vi "Expand Key.vi"(1 "Mode (auto)":enum16{"128", "192", "256", "auto"}(ring)=enum."auto", 7 "Key":u32[](array[numeric])=[49, 0, 0, 0, 0, 0, 0, 0, 0, 0, 0, 0, 0, 0, 0, 0, 0, 0, 0, 0, 0, 0, 0, 0, 0, 0, 0, 0, 0, 0, 0, 0], 11 "error in":errorcluster) -> (8 "Expanded Key":u32[](array[numeric]), 15 "error out":errorcluster)   [LabVIEW 2020, in "Library Commun.lvlib" / "Advanced Encryption Standard (AES).lvlib"]
doc: "The function KeyExpansion() supplies a much expanded (and transformed) key for use by the AddRoundKey() function in the main AES algorithm. In the case of the AES, there are a number of rounds, each needing its own key, so the actual key is ''stretched out'' and transformed to give portions of key for each round. This is the key expansion.\n\n<inline>"
uses:
  Advanced Encryption Standard (AES).lvlib
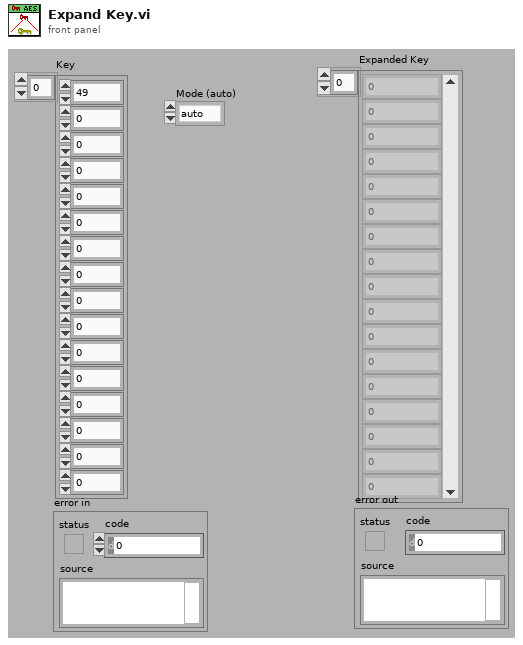
[diagram p1: front panel]
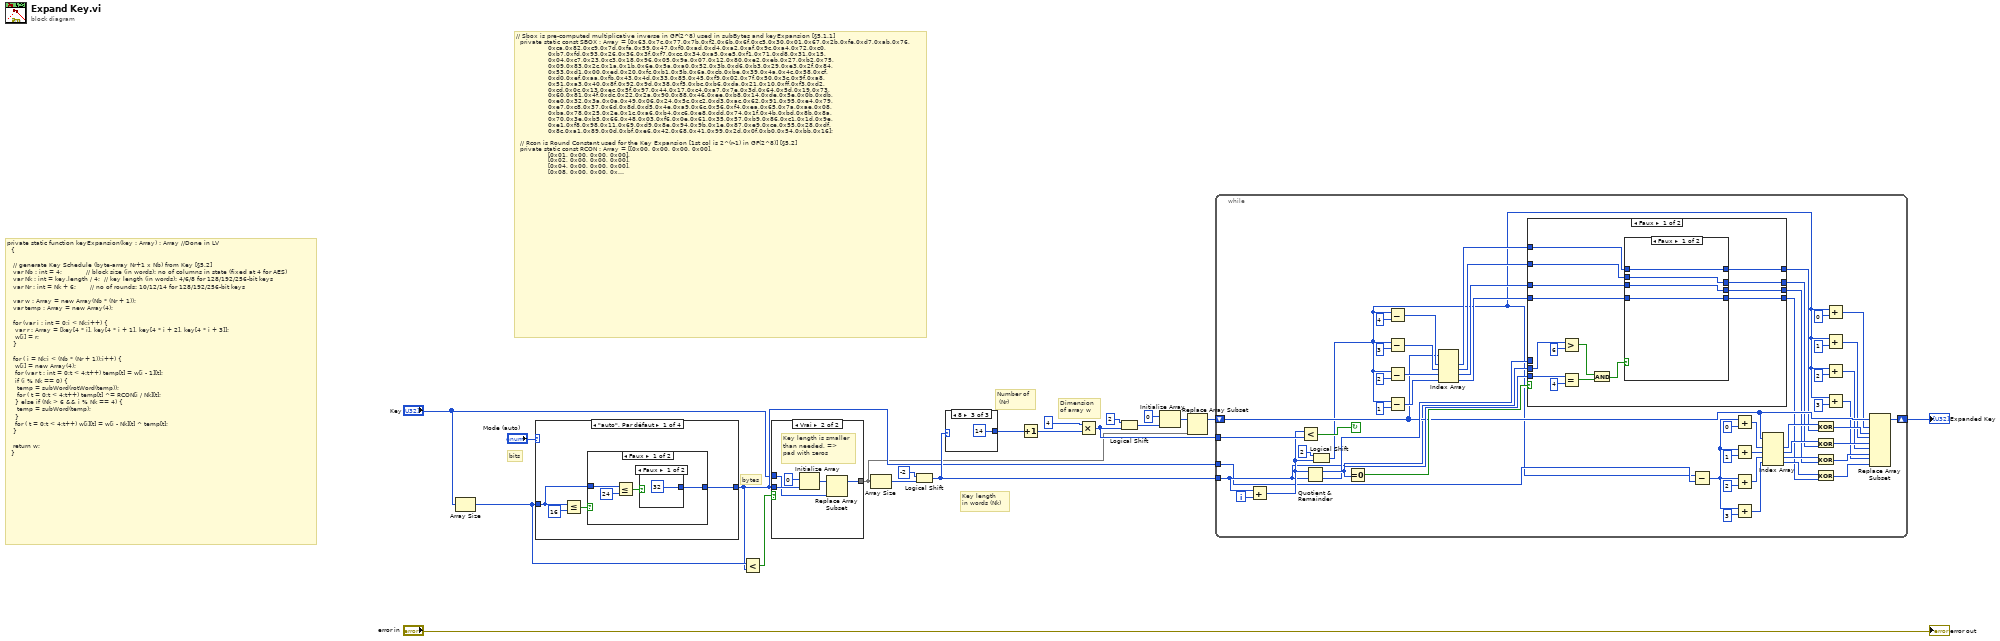
[diagram p0: block diagram]
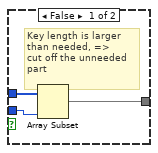
[diagram p2: hidden frame]
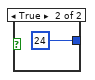
[diagram p3: hidden frame]
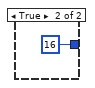
[diagram p4: hidden frame]
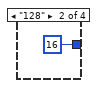
[diagram p5: hidden frame]
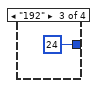
[diagram p6: hidden frame]
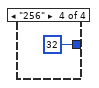
[diagram p7: hidden frame]
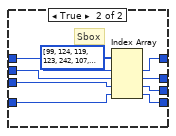
[diagram p8: hidden frame]
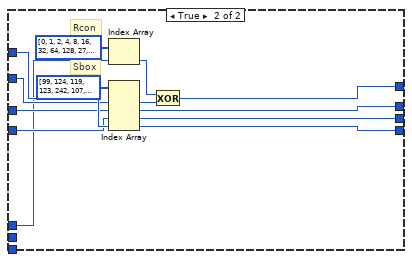
[diagram p9: hidden frame]
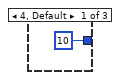
[diagram p10: hidden frame]
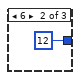
[diagram p11: hidden frame]
diagram:
  # "// Sbox is pre-computed multiplicative inverse in GF(2^8) used in subBytes and keyExpansion [§5.1.1]\n\t\tprivate static const SBOX : Array = [0x63,0x7c,0x77,0x7b,0xf2,0x6b,0x6f,0xc5,0x30,0x01,0x67,0x2b,0xfe,0xd7,0xab,0x76,\n\t\t\t             0xca,0x82,0xc9,0x7d,0xfa,0x59,0x47,0xf0,0xad,0xd4,0xa2,0xaf,0x9c,0xa4,0x72,0xc0,\n\t\t\t             0xb7,0xfd,0x93,0x26,0x36,0x3f,0xf7,0xcc,0x34,0xa5,0xe5,0xf1,0x71,0xd8,0x31,0x15,\n\t\t\t             0x04,0xc7,0x23,0xc3,0x18,0x96,0x05,0x9a,0x07,0x12,0x80,0xe2,0xeb,0x27,0xb2,0x75,\n\t\t\t             0x09,0x83,0x2c,0x1a,0x1b,0x6e,0x5a,0xa0,0x52,0x3b,0xd6,0xb3,0x29,0xe3,0x2f,0x84,\n\t\t\t             0x53,0xd1,0x00,0xed,0x20,0xfc,0xb1,0x5b,0x6a,0xcb,0xbe,0x39,0x4a,0x4c,0x58,0xcf,\n\t\t\t             0xd0,0xef,0xaa,0xfb,0x43,0x4d,0x33,0x85,0x45,0xf9,0x02,0x7f,0x50,0x3c,0x9f,0xa8,\n\t\t\t             0x51,0xa3,0x40,0x8f,0x92,0x9d,0x38,0xf5,0xbc,0xb6,0xda,0x21,0x10,0xff,0xf3,0xd2,\n\t\t\t             0xcd,0x0c,0x13,0xec,0x5f,0x97,0x44,0x17,0xc4,0xa7,0x7e,0x3d,0x64,0x5d,0x19,0x73,\n\t\t\t             0x60,0x81,0x4f,0xdc,0x22,0x2a,0x90,0x88,0x46,0xee,0xb8,0x14,0xde,0x5e,0x0b,0xdb,\n\t\t\t             0xe0,0x32,0x3a,0x0a,0x49,0x06,0x24,0x5c,0xc2,0xd3,0xac,0x62,0x91,0x95,0xe4,0x79,\n\t\t\t             0xe7,0xc8,0x37,0x6d,0x8d,0xd5,0x4e,0xa9,0x6c,0x56,0xf4,0xea,0x65,0x7a,0xae,0x08,\n\t\t\t             0xba,0x78,0x25,0x2e,0x1c,0xa6,0xb4,0xc6,0xe8,0xdd,0x74,0x1f,0x4b,0xbd,0x8b,0x8a,\n\t\t\t             0x70,0x3e,0xb5,0x66,0x48,0x03,0xf6,0x0e,0x61,0x35,0x57,0xb9,0x86,0xc1,0x1d,0x9e,\n\t\t\t             0xe1,0xf8,0x98,0x11,0x69,0xd9,0x8e,0x94,0x9b,0x1e,0x87,0xe9,0xce,0x55,0x28,0xdf,\n\t\t\t             0x8c,0xa1,0x89,0x0d,0xbf,0xe6,0x42,0x68,0x41,0x99,0x2d,0x0f,0xb0,0x54,0xbb,0x16];\n\n\t\t// Rcon is Round Constant used for the Key Expansion [1st col is 2^(r-1) in GF(2^8)] [§5.2]\n\t\tprivate static const RCON : Array = [[0x00, 0x00, 0x00, 0x00],\n\t\t\t             [0x01, 0x00, 0x00, 0x00],\n\t\t\t             [0x02, 0x00, 0x00, 0x00],\n\t\t\t             [0x04, 0x00, 0x00, 0x00],\n\t\t\t             [0x08, 0x00, 0x00, 0x00],\n\t\t\t             [0x10, 0x00, 0x00, 0x00],\n\t\t\t             [0x20, 0x00, 0x00, 0x00],\n\t\t\t             [0x40, 0x00, 0x00, 0x00],\n\t\t\t             [0x80, 0x00, 0x00, 0x00],\n\t\t\t             [0x1b, 0x00, 0x00, 0x00],\n\t\t\t             [0x36, 0x00, 0x00, 0x00]];"
  # "private static function keyExpansion(key : Array) : Array //Done in LV\n\t\t{  \n\t\t\t\n\t\t\t// generate Key Schedule (byte-array Nr+1 x Nb) from Key [§5.2]\n\t\t\tvar Nb : int = 4;            // block size (in words): no of columns in state (fixed at 4 for AES)\n\t\t\tvar Nk : int = key.length / 4;  // key length (in words): 4/6/8 for 128/192/256-bit keys\n\t\t\tvar Nr : int = Nk + 6;       // no of rounds: 10/12/14 for 128/192/256-bit keys\n\n\t\t\tvar w : Array = new Array(Nb * (Nr + 1));\n\t\t\tvar temp : Array = new Array(4);\n\t\t\t\n\t\t\tfor (var i : int = 0;i < Nk;i++) {\n\t\t\t\tvar r : Array = [key[4 * i], key[4 * i + 1], key[4 * i + 2], key[4 * i + 3]];\n\t\t\t\tw[i] = r;\n\t\t\t}\n\t\t\t\n\t\t\tfor ( i = Nk;i < (Nb * (Nr + 1));i++) {\n\t\t\t\tw[i] = new Array(4);\n\t\t\t\tfor (var t : int = 0;t < 4;t++) temp[t] = w[i - 1][t];\n\t\t\t\tif (i % Nk == 0) {\n\t\t\t\t\ttemp = subWord(rotWord(temp));\n\t\t\t\t\tfor ( t = 0;t < 4;t++) temp[t] ^= RCON[i / Nk][t];\n\t\t\t\t} else if (Nk > 6 && i % Nk == 4) {\n\t\t\t\t\ttemp = subWord(temp);\n\t\t\t\t}\n\t\t\t\tfor ( t = 0;t < 4;t++) w[i][t] = w[i - Nk][t] ^ temp[t];\n\t\t\t}\n\t\t\t\n\t\t\treturn w;\n\t\t}"
  # "Dimension \nof array w"
  # "Number of\n (Nr)"
  # "Key length \nin words (Nk)"
  # "bytes"
  # "bits"
  n1 = Array Size(array="Key") -> (size(s)=w7:i32)
  n2 = case shown="\"auto\", Par défaut" "Mode (auto)" {
    tunnel: w7 -> [w21 _ _ _]
    tunnel: [w22 16 24 32] -> w5
    frame "auto", Default {
      n3 = Less Or Equal?(x=w21, y=16) -> (x <= y?=w23:bool)
      n4 = case shown="Faux" w23 {
        tunnel: [w25 16] -> w22
        tunnel: w21 -> [w28 _]
        frame False {
          n5 = Less Or Equal?(x=w28, y=24) -> (x <= y?=w26:bool)
          n6 = case shown="Faux" w26 {
            tunnel: [32 ("y") 24 ("y")] -> w25
            frame False {
            }
            frame True {
            }
          }
        }
        frame True {
        }
      }
    }
    frame "128" {
    }
    frame "192" {
    }
    frame "256" {
    }
  }
  n7 = Less?(x=w7, y=w5) -> (x < y?=w6:bool)
  n8 = case shown="Vrai" w6 {
    tunnel: "Key" -> [w37 w38]
    tunnel: w5 -> [w36 w42]
    tunnel: [w35 w40] -> w4
    frame False {
      # "Key length is larger\nthan needed, =>\ncut off the unneeded\npart"
      n9 = Array Subset(array=w37, length=w36) -> (w35:u32[])  [unwired: 1 in]
    }
    frame True {
      # "Key length is smaller\nthan needed, =>\npad with zeros"
      n10 = Initialize Array(u32 0, w42) -> (w41:u32[])
      n11 = Replace Array Subset(array=w41, new element=w38) -> (w40:u32[])  [unwired: 1 in]
    }
  }
  n12 = Array Size(array=w4) -> (size(s)=w9:i32)
  n13 = Logical Shift(y=i8 -2, x=w9) -> (x << y=w16:i32)
  n14 = case shown="8" w16 {
    tunnel: [10 12 14] -> w19
    frame 4, Default {
    }
    frame 6 {
    }
    frame 8 {
    }
  }
  n15 = Increment(x=w19) -> (x+1=w18:i32)
  n16 = Multiply(x=4, y=w18) -> (x*y=w12:i32)
  n17 = Logical Shift(y=i8 2, x=w12) -> (x << y=w13:i32)
  n18 = Initialize Array(u32 0 ("element"), w13) -> (w11:u32[])
  n19 = Replace Array Subset(array=w11, new element=w4) -> (w10:u32[])  [unwired: 1 in]
  n20 = while {
    tunnel: w12 -> [w98]
    tunnel: w16 -> [w78]
    shift-right: [w55] -> w2
    shift-left: w10 -> [w79]
    tunnel: w5 -> [w77]
    i -> [w99]
    stop <- w97 continue-if-true
    n21 = Add(x=w78, y=w99) -> (x+y=w81:i32)
    n22 = Less?(x=w81, y=w98) -> (x < y?=w97:bool)
    n23 = Quotient & Remainder(x=w81, y=w78) -> (x-y*floor(x/y)=w86:i32, floor(x/y)=w80:i32)
    n24 = Logical Shift(y=i8 2, x=w81) -> (x << y=w50:i32)
    n25 = Equal To 0?(x=w86) -> (x = 0?=w87:bool)
    n26 = Subtract(x=w50, y=4) -> (x-y=w91:i32)
    n27 = Subtract(x=w50, y=3) -> (x-y=w90:i32)
    n28 = Subtract(x=w50, y=2) -> (x-y=w89:i32)
    n29 = Subtract(x=w50, y=1) -> (x-y=w88:i32)
    n30 = Index Array(array=w79, index #1=w91, index #2=w90, index #3=w89, index #4=w88) -> (element #1=w85:u32, element #2=w84:u32, element #3=w83:u32, element #4=w82:u32)
    n31 = case shown="Faux" w87 {
      tunnel: w78 -> [w114 _]
      tunnel: w86 -> [w112 _]
      tunnel: w85 -> [w107 w140]
      tunnel: w84 -> [w106 w139]
      tunnel: w83 -> [w105 w138]
      tunnel: w82 -> [w104 w137]
      tunnel: w80 -> [_ w136]
      tunnel: [w103 w133] -> w59
      tunnel: [w102 w132] -> w58
      tunnel: [w101 w131] -> w57
      tunnel: [w100 w130] -> w56
      frame False {
        n32 = Greater?(x=w114, y=6) -> (0:w110:bool)
        n33 = Equal?(x=w112, y=4) -> (x = y?=w109:bool)
        n34 = And(x=w110, y=w109) -> (x .and. y?=w108:bool)
        n35 = case shown="Faux" w108 {
          tunnel: w107 -> [w118 w127]
          tunnel: w106 -> [w117 w126]
          tunnel: w105 -> [w116 w125]
          tunnel: w104 -> [w115 w124]
          tunnel: [w118 w123] -> w103
          tunnel: [w117 w122] -> w102
          tunnel: [w116 w121] -> w101
          tunnel: [w115 w120] -> w100
          frame False {
          }
          frame True {
            # "Sbox"
            n36 = Index Array(array=u32[] [99, 124, 119, 123, 242, 107, 111, 197, 48, 1, 103, 43, 254, 215, 171, 118, 202, 130, 201, 125, 250, 89, 71, 240, 173, 212, 162, 175, 156, 164, 114, 192, 183, 253, 147, 38, 54, 63, 247, 204, 52, 165, 229, 241, 113, 216, 49, 21, 4, 199, 35, 195, 24, 150, 5, 154, 7, 18, 128, 226, 235, 39, 178, 117, 9, 131, 44, 26, 27, 110, 90, 160, 82, 59, 214, 179, 41, 227, 47, 132, 83, 209, 0, 237, 32, 252, 177, 91, 106, 203, 190, 57, 74, 76, 88, 207, 208, 239, 170, 251, 67, 77, 51, 133, 69, 249, 2, 127, 80, 60, 159, 168, 81, 163, 64, 143, 146, 157, 56, 245, 188, 182, 218, 33, 16, 255, 243, 210, 205, 12, 19, 236, 95, 151, 68, 23, 196, 167, 126, 61, 100, 93, 25, 115, 96, 129, 79, 220, 34, 42, 144, 136, 70, 238, 184, 20, 222, 94, 11, 219, 224, 50, 58, 10, 73, 6, 36, 92, 194, 211, 172, 98, 145, 149, 228, 121, 231, 200, 55, 109, 141, 213, 78, 169, 108, 86, 244, 234, 101, 122, 174, 8, 186, 120, 37, 46, 28, 166, 180, 198, 232, 221, 116, 31, 75, 189, 139, 138, 112, 62, 181, 102, 72, 3, 246, 14, 97, 53, 87, 185, 134, 193, 29, 158, 225, 248, 152, 17, 105, 217, 142, 148, 155, 30, 135, 233, 206, 85, 40, 223, 140, 161, 137, 13, 191, 230, 66, 104, 65, 153, 45, 15, 176, 84, 187, 22] ("Sbox"), index #1=w127, index #2=w126, index #3=w125, index #4=w124) -> (element #1=w123:u32, element #2=w122:u32, element #3=w121:u32, element #4=w120:u32)
          }
        }
      }
      frame True {
        # "Sbox"
        # "Rcon"
        n37 = Index Array(array=u32[] [0, 1, 2, 4, 8, 16, 32, 64, 128, 27, 54] ("Rcon"), index=w136) -> (element=w135:u32)
        n38 = Index Array(array=u32[] [99, 124, 119, 123, 242, 107, 111, 197, 48, 1, 103, 43, 254, 215, 171, 118, 202, 130, 201, 125, 250, 89, 71, 240, 173, 212, 162, 175, 156, 164, 114, 192, 183, 253, 147, 38, 54, 63, 247, 204, 52, 165, 229, 241, 113, 216, 49, 21, 4, 199, 35, 195, 24, 150, 5, 154, 7, 18, 128, 226, 235, 39, 178, 117, 9, 131, 44, 26, 27, 110, 90, 160, 82, 59, 214, 179, 41, 227, 47, 132, 83, 209, 0, 237, 32, 252, 177, 91, 106, 203, 190, 57, 74, 76, 88, 207, 208, 239, 170, 251, 67, 77, 51, 133, 69, 249, 2, 127, 80, 60, 159, 168, 81, 163, 64, 143, 146, 157, 56, 245, 188, 182, 218, 33, 16, 255, 243, 210, 205, 12, 19, 236, 95, 151, 68, 23, 196, 167, 126, 61, 100, 93, 25, 115, 96, 129, 79, 220, 34, 42, 144, 136, 70, 238, 184, 20, 222, 94, 11, 219, 224, 50, 58, 10, 73, 6, 36, 92, 194, 211, 172, 98, 145, 149, 228, 121, 231, 200, 55, 109, 141, 213, 78, 169, 108, 86, 244, 234, 101, 122, 174, 8, 186, 120, 37, 46, 28, 166, 180, 198, 232, 221, 116, 31, 75, 189, 139, 138, 112, 62, 181, 102, 72, 3, 246, 14, 97, 53, 87, 185, 134, 193, 29, 158, 225, 248, 152, 17, 105, 217, 142, 148, 155, 30, 135, 233, 206, 85, 40, 223, 140, 161, 137, 13, 191, 230, 66, 104, 65, 153, 45, 15, 176, 84, 187, 22] ("Sbox"), index #1=w139, index #2=w138, index #3=w137, index #4=w140) -> (element #1=w134:u32, element #2=w132:u32, element #3=w131:u32, element #4=w130:u32)
        n39 = Exclusive Or(1:w134, 2:w135) -> (0:w133:u32)
      }
    }
    n40 = Subtract(x=w50, y=w77) -> (x-y=w76:i32)
    n41 = Add(x=w76, y=0) -> (x+y=w71:i32)
    n42 = Add(x=w76, y=1) -> (x+y=w70:i32)
    n43 = Add(x=w76, y=2) -> (x+y=w69:i32)
    n44 = Add(x=w76, y=3) -> (x+y=w68:i32)
    n45 = Index Array(array=w79, index #1=w71, index #2=w70, index #3=w69, index #4=w68) -> (element #1=w67:u32, element #2=w66:u32, element #3=w65:u32, element #4=w64:u32)
    n46 = Exclusive Or(1:w59, 2:w67) -> (0:w63:u32)
    n47 = Exclusive Or(1:w58, 2:w66) -> (0:w62:u32)
    n48 = Exclusive Or(1:w57, 2:w65) -> (0:w61:u32)
    n49 = Exclusive Or(1:w56, 2:w64) -> (0:w60:u32)
    n50 = Add(x=w50, y=0) -> (x+y=w49:i32)
    n51 = Add(x=w50, y=1) -> (x+y=w48:i32)
    n52 = Add(x=w50, y=2) -> (x+y=w47:i32)
    n53 = Add(x=w50, y=3) -> (x+y=w46:i32)
    n54 = Replace Array Subset(array=w79, new element #1=w63, index #1=w49, new element #2=w62, index #2=w48, new element #3=w61, index #3=w47, new element #4=w60, index #4=w46) -> (w55:u32[])
  }
  "Expanded Key" <- w2
  "error out" <- "error in"
